vi "Process Request.vi"(8 "error in":errorcluster, 10 "Requested":bool, 11 "Delay Timer in":refnum<class "Output Timer.lvclass">) -> (0 "error out":errorcluster, 2 "Returned":bool, 3 "Delay Timer out":refnum<class "Output Timer.lvclass">)   [LabVIEW 2013, in "Output Timer.lvclass"]
doc: "This VI takes a boolean input (<b>Requested</b>) and checks to see if the class is in a state to acknowledge the value. If it is possible, the instance of the Output Timer class will acknowledge the request and switch the value. If not, then the value <b>Requested</b> will not match the value <b>Returned</b>.\n\nThere will be a mismatch if the caller attempts to change the value from FALSE to TRUE without sufficient time passing. The amount of time should be set bu the caller and is located in the class property <b>Delay</b>. This VI compares the this property with the amount of time passed since the last switch from TRUE to FALSE stored in the property <b>Last Switch</b> of the current instance of the Output Timer class. At startup, the initial switch state is FALSE and the <b>Last Switch</b> property is defaulted to 0."
uses:
  Output Timer.lvclass
  Output Timer.lvclass/Output Timer.ctl
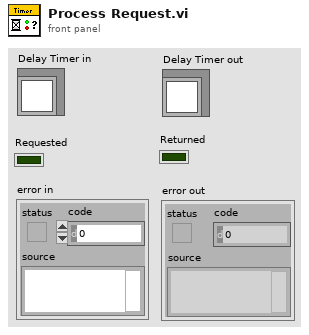
[diagram p1: front panel]
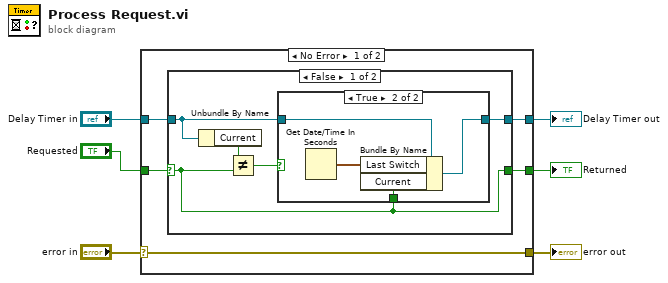
[diagram p0: block diagram]
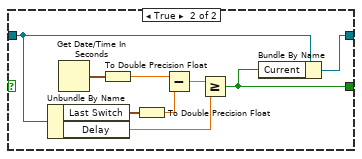
[diagram p3: hidden frame]
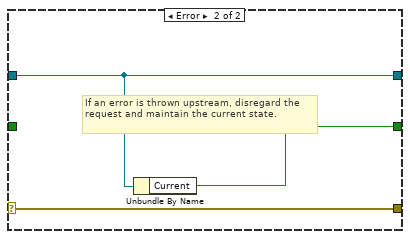
[diagram p4: hidden frame]
diagram:
  n1 = case shown="No Error" "error in" {
    selector: "error in" -> [w11 w33]
    tunnel: [w11 w33] -> w5
    tunnel: [w7 w32] -> w3
    tunnel: "Delay Timer in" -> [w8 w32]
    tunnel: "Requested" -> [w10 _]
    tunnel: [w9 w31] -> w1
    frame No Error {
      n2 = case shown="False" w10 {
        selector: w10 -> [w13 _]
        tunnel: [w13 w22] -> w9
        tunnel: w8 -> [w15 w24]
        tunnel: [w16 w23] -> w7
        frame False {
          n3 = Unbundle By Name(w15) -> ("Current"=w14:bool)
          n4 = Not Equal?(x=w14, y=w13) -> (x != y?=w12:bool)
          n5 = case shown="True" w12 {
            tunnel: [w17 w21] -> w16
            tunnel: w15 -> [w17 w19]
            tunnel: w13 -> [_ w18]
            frame False {
            }
            frame True {
              n6 = Get Date/Time In Seconds() -> (seconds since 1Jan1904=w20:timestamp)
              n7 = Bundle By Name(cluster=w19, "Last Switch"=w20, "Current"=w18) -> (w21:refnum<class "Output Timer.lvclass">)
            }
          }
        }
        frame True {
          n8 = Unbundle By Name(w24) -> ("Last Switch"=w28:timestamp, "Delay"=w25:dbl)
          n9 = Get Date/Time In Seconds() -> (seconds since 1Jan1904=w30:timestamp)
          n10 = To Double Precision Float(number=w30) -> (double precision float=w29:dbl)
          n11 = To Double Precision Float(number=w28) -> (double precision float=w27:dbl)
          n12 = Subtract(x=w29, y=w27) -> (x-y=w26:dbl)
          n13 = Greater Or Equal?(x=w26, y=w25) -> (x >= y?=w22:bool)
          n14 = Bundle By Name(cluster=w24, "Current"=w22) -> (w23:refnum<class "Output Timer.lvclass">)
        }
      }
    }
    frame Error {
      # "If an error is thrown upstream, disregard the request and maintain the current state."
      n15 = Unbundle By Name(w32) -> ("Current"=w31:bool)
    }
  }
  "error out" <- w5
  "Delay Timer out" <- w3
  "Returned" <- w1
